vi "Validate Sequence.vi"(11 "Auton Sequence":T1[](array[typedef])) -> (2 "Command Name":string, 3 "Sequence Ok?":bool)   [LabVIEW 2017]
uses:
  Typedef/Single Sequence.ctl
  Typedef/Sequence Command.ctl
  Typedef/Plate Arrangement.ctl
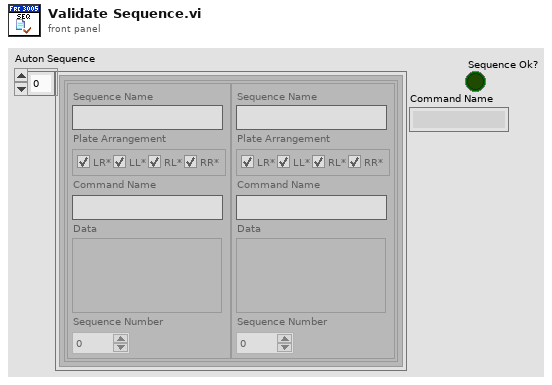
[diagram p1: front panel]
types:
  T1 = typedef "Single Sequence.ctl" = cluster{"Sequence Array":T2[]}
  T2 = typedef "Sequence Command.ctl" = cluster{"Sequence Name":string, "Plate Arrangement":T3, "Command Name":string, "Data":variant, "Sequence Number":u32}
  T3 = typedef "Plate Arrangement.ctl" = cluster{"LR*":bool, "LL*":bool, "RL*":bool, "RR*":bool}
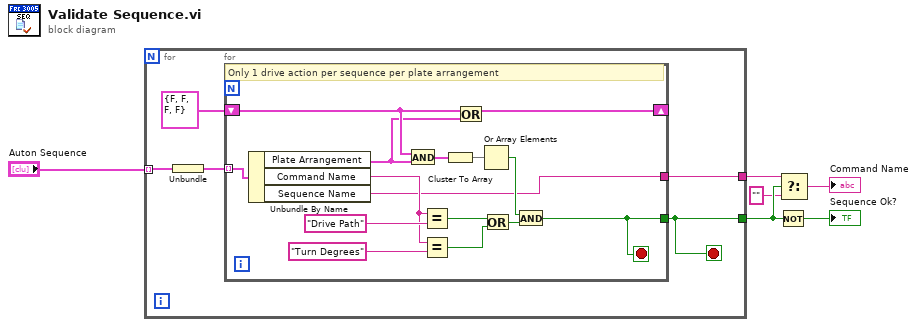
[diagram p0: block diagram]
diagram:
  n1 = for {
    tunnel: "Auton Sequence" -> [w11] mode=indexing
    tunnel: [w8] -> w4
    tunnel: [w7] -> w3
    stop <- w8 stop-if-true
    n2 = Unbundle(w11) -> ("Sequence Array"=w10:T2[])
    n3 = for {
      tunnel: w10 -> [w26] mode=indexing
      shift-right: [w23] -> _
      shift-left: T3 {"LR*"=FALSE, "LL*"=FALSE, "RL*"=FALSE, "RR*"=FALSE} ("Plate Arrangement") -> [w25]
      tunnel: [w14] -> w8
      tunnel: [w12] -> w7
      stop <- w14 stop-if-true
      # "Only 1 drive action per sequence per plate arrangement"
      n4 = Unbundle By Name(w26) -> ("Plate Arrangement"=w24:T3, "Command Name"=w13:string, "Sequence Name"=w12:string)
      n5 = And(x=w25, y=w24) -> (x .and. y?=w22:T3)
      n6 = Equal?(x=w13, y="Drive Path") -> (x = y?=w15:bool)
      n7 = Equal?(x=w13, y="Turn Degrees") -> (x = y?=w16:bool)
      n8 = Cluster To Array(cluster=w22) -> (array=w21:bool[])
      n9 = Or(x=w25, y=w24) -> (x .or. y?=w23:T3)
      n10 = Or Array Elements(Boolean array=w21) -> (logical OR=w20:bool)
      n11 = Or(x=w15, y=w16) -> (x .or. y?=w18:bool)
      n12 = And(x=w20, y=w18) -> (x .and. y?=w14:bool)
    }
  }
  n13 = Not(x=w4) -> (.not. x?=→"Sequence Ok?":bool)
  n14 = Select(t=w3, s=w4, f="") -> (s? t:f=→"Command Name":string)
